vi "Auto Drive Calibrations.vi"() -> ()   [LabVIEW 2016]
panel:
  in  "Auto Drive Calibrations File Location":path=path "C:/ni-rt/startup/AutoDriveCalibrations.txt"
  out "PID Tracking":T1(graph)={"Goal"=0.0, "Process Variable"=648.45703125, "Max Ouput"=-300.0, -648.45703125, -3242.28515625, 0.0, 0.0}
  out "Drive to Encoders Derivative Gain":dbl
  out "Drive to Encoders Proportional Gain":dbl=0.6
  out "Drive to Encoders Integral Gain":dbl
  out "Drive Time with IMU Derivative Gain":dbl=3.0
  out "Drive Time with IMU Proportional Gain":dbl=4.0
  out "Drive Time with IMU Integral Gain":dbl
  out "Auto Drive":bool
  out "Right Auto Drive Derivative Gain":dbl
  out "Right Auto Drive Feed-Forward Gain":dbl=0.45
  out "Right Auto Drive Proportional Gain":dbl=0.6
  out "Right Auto Drive Integral Gain":dbl
  out "Left Auto Drive Derivative Gain":dbl
  out "Left Auto Drive Feed-Forward Gain":dbl=0.42
  out "Left Auto Drive Proportional Gain":dbl=0.6
  out "Left Auto Drive Integral Gain":dbl
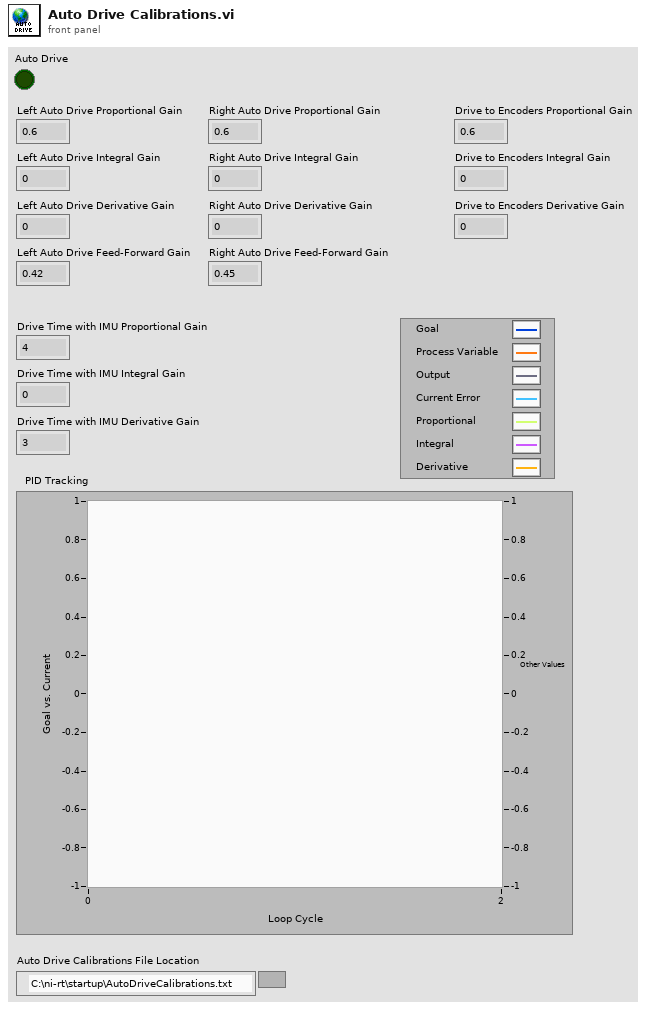
[diagram p1: front panel]
types:
  T1 = cluster{"Goal":dbl, "Process Variable":dbl, "Max Ouput":dbl, dbl, dbl, dbl, dbl}
diagram:
